vi "Example_PortToggle.vi"() -> ()   [LabVIEW 2021, in "BrainStem2_LabVIEW_Library.lvlib"]
uses:
  BrainStem2_LabVIEW_Library.lvlib
panel:
  out "Port 3 Current":u32
  out "Port 3 Voltage":u32
  out "Port 2 Current":u32
  out "Port 2 Voltage":u32
  out "Port 1 Current":u32
  out "Port 1 Voltage":u32
  out "Port 0 Current":u32
  out "Port 0 Voltage":u32
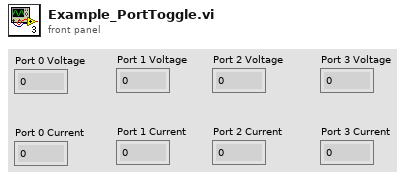
[diagram p1: front panel]
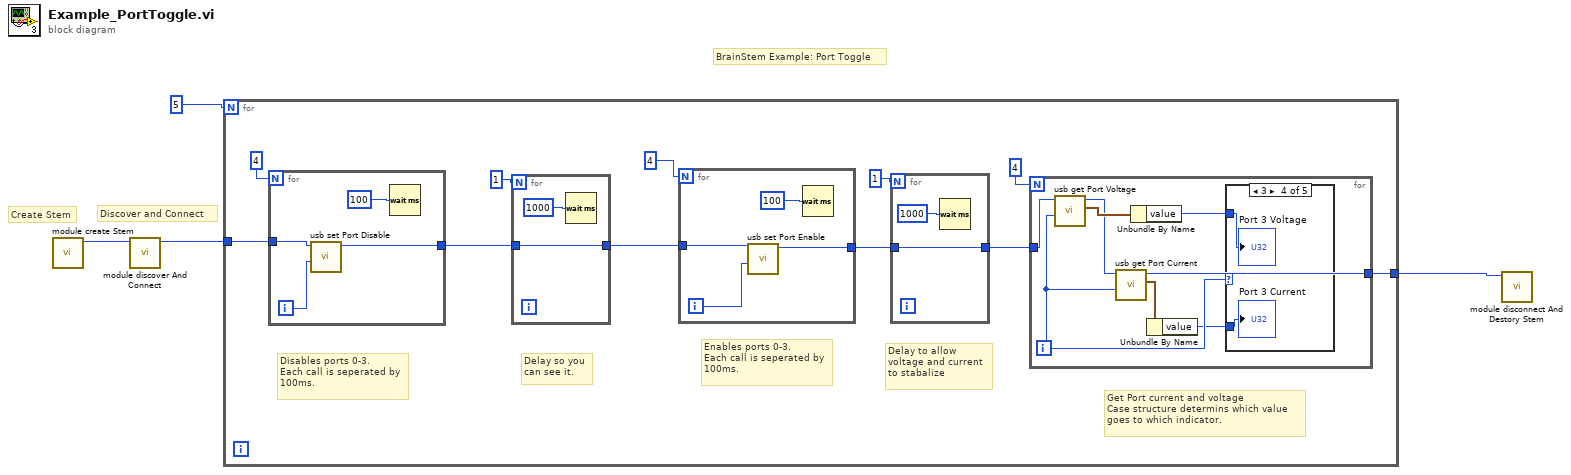
[diagram p0: block diagram]
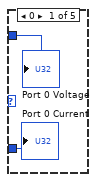
[diagram p2: hidden frame]
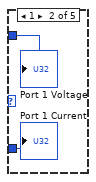
[diagram p3: hidden frame]
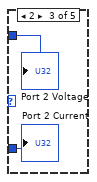
[diagram p4: hidden frame]
diagram:
  # "Discover and Connect"
  # "Create Stem"
  # "BrainStem Example: Port Toggle"
  n1 = call "module create Stem.vi"() -> ("id out"=w4:u32)  [unwired: 9 in, 2 out]
  n2 = call "module discover And Connect.vi"("id"=w4) -> ("id out"=w3:u32)  [unwired: 8 in, 2 out]
  n3 = for {
    N: 5 -> [_]
    tunnel: w3 -> [w11]
    tunnel: [w5] -> w2
    # "Get Port current and voltage\nCase structure determins which value\ngoes to which indicator."
    # "Delay to allow\nvoltage and current\nto stabalize"
    # "Enables ports 0-3.\nEach call is seperated by\n100ms."
    # "Delay so you\ncan see it."
    # "Disables ports 0-3.\nEach call is seperated by\n100ms."
    n4 = for {
      N: 4 -> [_]
      tunnel: w11 -> [w41]
      tunnel: [w40] -> w9
      i -> [w42]
      n5 = call "usb set Port Disable.vi"("channel"=w42, "id"=w41) -> ("id out"=w40:u32)  [unwired: 7 in, 2 out]
      n6 = Wait (ms)(milliseconds to wait=100) -> ()  [unwired: 1 out]
    }
    n7 = for {
      N: 1 -> [_]
      tunnel: [w32] -> w10
      tunnel: w9 -> [w32]
      n8 = Wait (ms)(milliseconds to wait=1000) -> ()  [unwired: 1 out]
    }
    n9 = for {
      N: 4 -> [_]
      tunnel: w10 -> [w37]
      tunnel: [w36] -> w7
      i -> [w38]
      n10 = call "usb set Port Enable.vi"("channel"=w38, "id"=w37) -> ("id out"=w36:u32)  [unwired: 7 in, 2 out]
      n11 = Wait (ms)(milliseconds to wait=100) -> ()  [unwired: 1 out]
    }
    n12 = for {
      N: 1 -> [_]
      tunnel: [w34] -> w8
      tunnel: w7 -> [w34]
      n13 = Wait (ms)(milliseconds to wait=1000) -> ()  [unwired: 1 out]
    }
    n14 = for {
      N: 4 -> [_]
      tunnel: w8 -> [w17]
      tunnel: [w16] -> w5
      i -> [w20]
      n15 = call "usb get Port Voltage.vi"("channel"=w20, "id"=w17) -> ("result out"=w23:cluster{"value":i32, "error":i32}, "id out"=w21:u32)  [unwired: 7 in, 1 out]
      n16 = call "usb get Port Current.vi"("channel"=w20, "id"=w21) -> ("result out"=w22:cluster{"value":i32, "error":i32}, "id out"=w16:u32)  [unwired: 7 in, 1 out]
      n17 = Unbundle By Name(w23) -> ("value"=w19:i32)
      n18 = Unbundle By Name(w22) -> ("value"=w18:i32)
      n19 = case shown="3" w20 {
        tunnel: w19 -> [w25 w27 w29 w31 _]
        tunnel: w18 -> [w24 w26 w28 w30 _]
        frame 0 {
          "Port 0 Voltage" <- w25
          "Port 0 Current" <- w24
        }
        frame 1 {
          "Port 1 Voltage" <- w27
          "Port 1 Current" <- w26
        }
        frame 2 {
          "Port 2 Voltage" <- w29
          "Port 2 Current" <- w28
        }
        frame 3 {
          "Port 3 Voltage" <- w31
          "Port 3 Current" <- w30
        }
        frame 4, Default {
        }
      }
    }
  }
  n20 = call "module disconnect And Destory Stem.vi"("id"=w2) -> ()  [unwired: 8 in, 3 out]
